vi "WPI_DashboardRetrieve NetworkTables2.vi"(8 "Docked Window":bool, 11 "DB Main Ref":refnum<vi>) -> (3 "Strings":T1)   [LabVIEW 2025]
uses:
  <vilib>/Rock Robotics/WPI/Dashboard/WPI_DashboardNTL Header Type.ctl
  <vilib>/Rock Robotics/WPI/Dashboard/WPI_DashboardLogging Global.vi
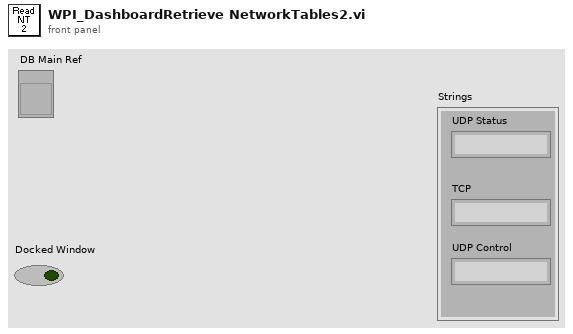
[diagram p1: front panel]
types:
  T1 = cluster{"UDP Status":string, "TCP":string, "UDP Control":string}
  T2 = typedef "WPI_DashboardNTL Header Type.ctl" = cluster{"Version":i32, "Duration (ms)":i32, "TimeStamp":timestamp, "Robot IP":string, "Displays":string[]}
  T3 = cluster{"Scale.Range:Minimum":dbl, dbl, "Scale.Range:Minimum":dbl, "Scale.Range:Minimum":dbl, "Scale.Range:Minimum":dbl}
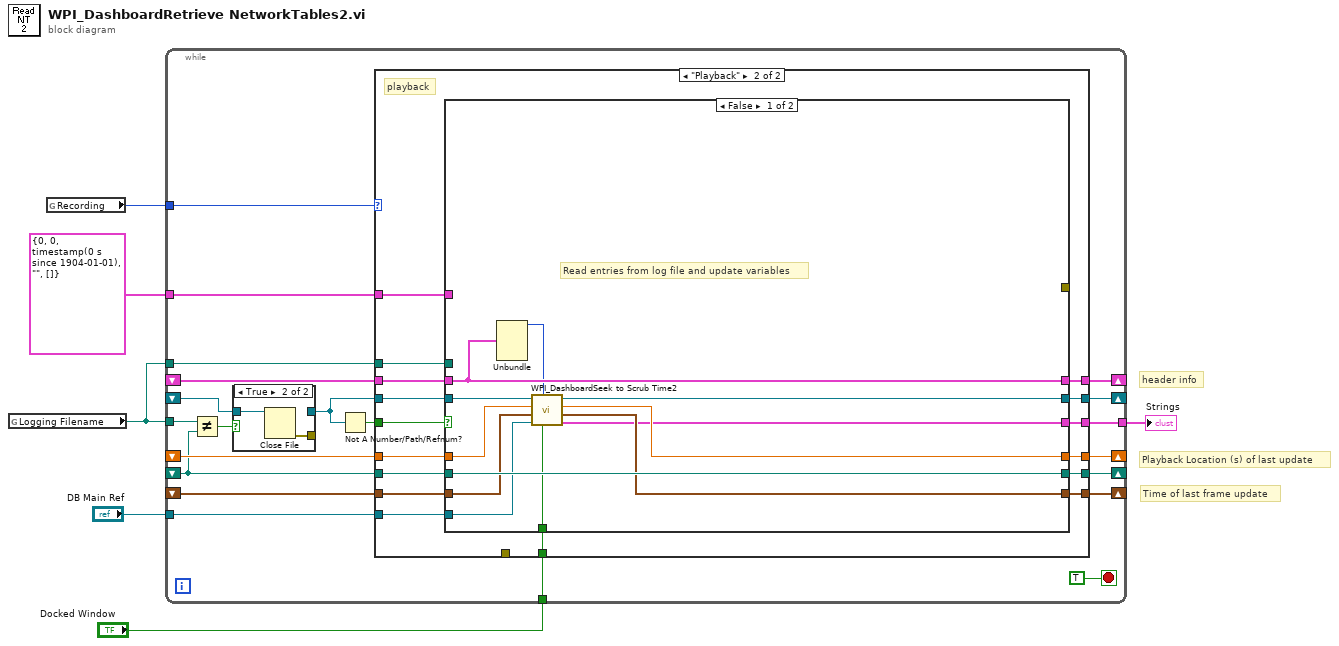
[diagram p0: block diagram]
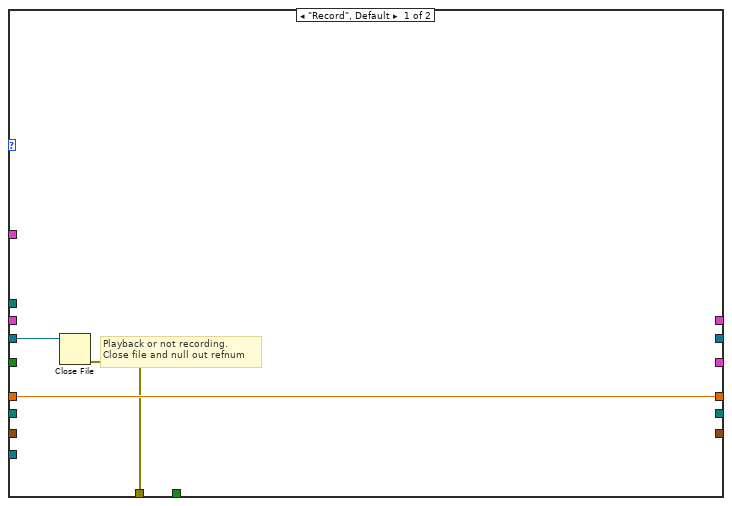
[diagram p3: hidden frame]
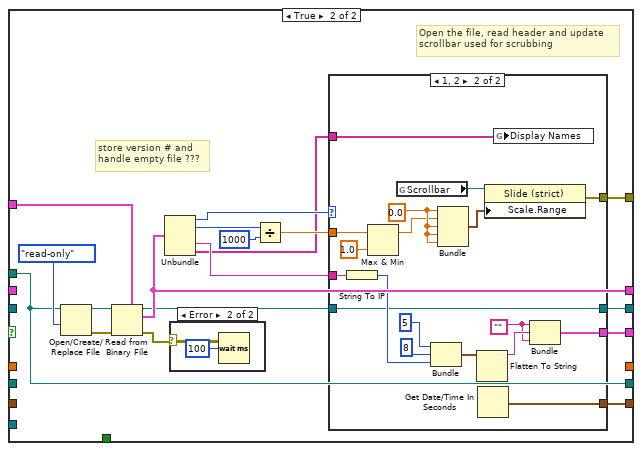
[diagram p4: hidden frame]
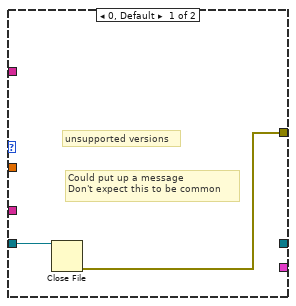
[diagram p5: hidden frame]
diagram:
  # "Time of last frame update"
  # "header info"
  # "Playback Location (s) of last update"
  n1 = global read "WPI_DashboardLogging Global.vi" "Logging Filename"() -> (w4:path)
  n2 = global read "WPI_DashboardLogging Global.vi" "Recording"() -> (w5:enum32{"Stop", "Record", "Playback"})
  n3 = while {
    shift-right: [w26] -> _
    shift-left: _ -> [w12]
    shift-right: [w24] -> _
    shift-left: _ -> [w23]
    shift-right: [w22] -> _
    shift-left: _ -> [w21]
    tunnel: T2 {"Version"=0, "Duration (ms)"=0, "TimeStamp"=timestamp(0 s since 1904-01-01), "Robot IP"="", "Displays"=[]} ("Header") -> [w20]
    shift-right: [w19] -> _
    shift-left: _ -> [w18]
    shift-right: [w16] -> _
    shift-left: _ -> [w15]
    tunnel: w5 -> [w9]
    tunnel: w4 -> [w17]
    tunnel: w4 -> [w11]
    tunnel: [w10] -> w1
    tunnel: "DB Main Ref" -> [w8]
    tunnel: "Docked Window" -> [w7]
    stop <- TRUE stop-if-true
    n4 = Not Equal?(x=w17, y=w15) -> (x != y?=w14:bool)
    n5 = case shown="True" w14 {
      tunnel: [w28 _] -> w13
      tunnel: w12 -> [w28 w30]
      tunnel: [_ w29] -> _
      frame False {
      }
      frame True {
        n6 = Close File(refnum=w30) -> (error out=w29:errorcluster)  [unwired: 1 in, 1 out]
      }
    }
    n7 = Not A Number/Path/Refnum?(number/path/refnum=w13) -> (NaN/Path/Refnum?=w25:bool)
    n8 = case shown="\"Playback\"" w9 {
      tunnel: [_ w49] -> w26
      tunnel: w13 -> [w33 w48]
      tunnel: w25 -> [_ w47]
      tunnel: [w32 w46] -> w24
      tunnel: w23 -> [w32 w45]
      tunnel: [_ w44] -> w22
      tunnel: w21 -> [_ w43]
      tunnel: w20 -> [_ w42]
      tunnel: [_ w41] -> w19
      tunnel: w18 -> [_ w40]
      tunnel: [_ w39] -> w16
      tunnel: w15 -> [_ w38]
      tunnel: w11 -> [_ w37]
      tunnel: [w31 _] -> _
      tunnel: [_ w36] -> w10
      tunnel: w8 -> [_ w35]
      tunnel: w7 -> [_ w34]
      frame "Record", Default {
        # "Playback or not recording.\nClose file and null out refnum"
        n9 = Close File(refnum=w33) -> (error out=w31:errorcluster)  [unwired: 1 in, 1 out]
      }
      frame "Playback" {
        # "playback"
        n10 = case shown="False" w47 {
          tunnel: [w55 w63] -> w49
          tunnel: w48 -> [w60 _]
          tunnel: [w54 _] -> w46
          tunnel: w45 -> [w59 _]
          tunnel: [w51 w76] -> w44
          tunnel: w43 -> [w51 _]
          tunnel: w42 -> [_ w75]
          tunnel: [w53 w72] -> w41
          tunnel: w40 -> [w58 _]
          tunnel: [w61 w71] -> w39
          tunnel: w38 -> [w61 _]
          tunnel: w37 -> [_ w71]
          tunnel: [_ w69] -> _
          tunnel: [w52 w66] -> w36
          tunnel: w35 -> [w57 _]
          tunnel: w34 -> [w56 _]
          frame False {
            # "Read entries from log file and update variables"
            n11 = Unbundle(w51) -> ("Version"=w50:i32)  [unwired: 4 out]
            n12 = call <vilib>:"WPI_DashboardSeek to Scrub Time2.vi"("Docked Window"=w56, "Version"=w50, "VI Refnum"=w57, "latest update tick"=w58, "TimeOffset (s)"=w59, "Byte Stream File in"=w60) -> ("Strings"=w52:T1, "ms tick out"=w53:timestamp, "TimeOffset (s) out"=w54:dbl, "Byte Stream File out"=w55:refnum<file>)  [unwired: 2 in]
          }
          frame True {
            # "store version # and\nhandle empty file ???"
            # "Open the file, read header and update\nscrollbar used for scrubbing"
            n13 = Open/Create/Replace File(file path (use dialog)=w71, access (0:read/write)=enum16{"read/write", "read-only", "write-only"}."read-only") -> (refnum out=w78:refnum<file>, error out=w77:errorcluster)  [unwired: 4 in, 1 out]
            n14 = Read from Binary File(5:w75, 8:w77, 11:w78) -> (0:w68:errorcluster, 2:w76:T2, 3:w64:refnum<file>)  [unwired: 3 in, 1 out]
            n15 = Unbundle(w76) -> ("Version"=w65:i32, "Duration (ms)"=w74:i32, "Robot IP"=w67:string, "Displays"=w62:string[])  [unwired: 1 out]
            n16 = case shown="Error" w68 {
              frame No Error {
              }
              frame Error {
                n17 = Wait (ms)(milliseconds to wait=u32 100) -> ()  [unwired: 1 out]
              }
            }
            n18 = Divide(x=w74, y=1000) -> (x/y=w70:dbl)
            n19 = case shown="1, 2" w65 {
              tunnel: [_ w98] -> w72
              tunnel: w70 -> [_ w96]
              tunnel: [w80 w92] -> w69
              tunnel: w67 -> [_ w91]
              tunnel: [_ w84] -> w66
              tunnel: w64 -> [w81 w83]
              tunnel: [_ w83] -> w63
              tunnel: w62 -> [_ w82]
              frame 0, Default {
                # "Could put up a message\nDon't expect this to be common"
                # "unsupported versions"
                n20 = Close File(refnum=w81) -> (error out=w80:errorcluster)  [unwired: 1 in, 1 out]
              }
              frame 1, 2 {
                w85 = ""
                w94 = 0.0 ("Scale.Range:Minimum")
                n21 = String To IP(1:w91) -> (0:w87:u32)
                n22 = Max & Min(x=w96, y=1.0 ("Scale.Range:Minimum")) -> (max(x,y)=w93:dbl)  [unwired: 1 out]
                n23 = global read "WPI_DashboardLogging Global.vi" "Scrollbar"() -> (w99:refnum<vi>)
                n24 = Bundle("index"=u16 5, "index"=u8 8, w87) -> (w89:cluster{"index":u16, "index":u8, u32})  [unwired: 1 in]
                n25 = Bundle("Scale.Range:Minimum"=w94, w93, "Scale.Range:Minimum"=w94, "Scale.Range:Minimum"=w94, "Scale.Range:Minimum"=w94) -> (w95:T3)  [unwired: 1 in]
                n26 = Flatten To String(anything=w89) -> (data string=w86:string)  [unwired: 3 in, 2 out]
                n27 = Get Date/Time In Seconds() -> (seconds since 1Jan1904=w98:timestamp)
                n28 = property class="Slide (strict)"(reference=w99, "Scale.Range"=w95) -> (error out=w92:errorcluster)  [unwired: 1 in, 1 out]
                n29 = global write "WPI_DashboardLogging Global.vi" "Display Names"(w82) -> ()
                n30 = Bundle(w85, "data string"=w86, w85) -> (w84:cluster{string, "data string":string, string})  [unwired: 1 in]
              }
            }
          }
        }
      }
    }
  }
  "Strings" <- w1
